vi "findChannelIndexes.vi"(8 "error in (no error)":errorcluster, 10 "index":i32, 11 "ScriptEventList in":refnum<class "ScriptEventList.lvclass">) -> (0 "error out":errorcluster, 1 "noneFound":bool, 2 "indexArray":i32[](array[numeric]), 3 "ScriptEventList out":refnum<class "ScriptEventList.lvclass">)   [LabVIEW 2009, in "Tools.lvlib" / "Scripting.lvlib" / "ScriptEventList.lvclass"]
uses:
  ScriptEventList.lvclass
  ScriptEventList.lvclass/ScriptEventList.ctl
  ScriptEvent.lvclass
  DatabaseHelpers/Database Objects/Channel/Channel.lvclass
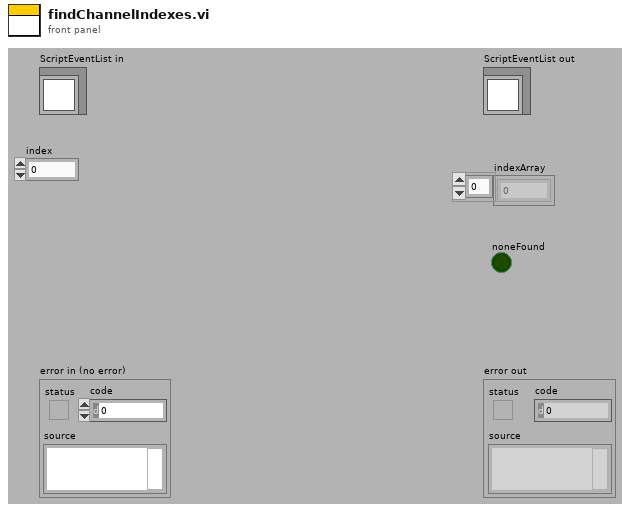
[diagram p1: front panel]
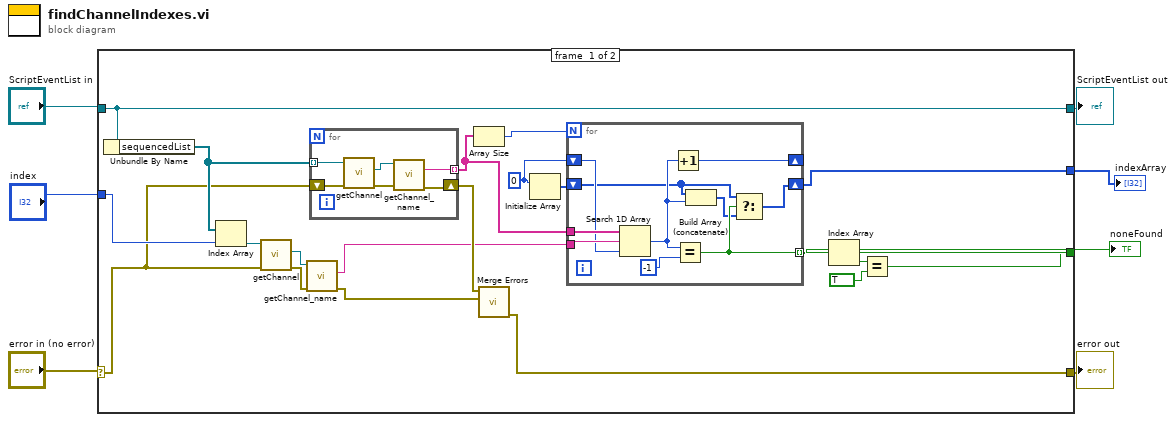
[diagram p0: block diagram]
diagram:
  n1 = case shown="No Error" "error in (no error)" {
    selector: "error in (no error)" -> [w21 w45]
    tunnel: [w23 w45] -> w1
    tunnel: [w27 w44] -> w4
    tunnel: "ScriptEventList in" -> [w27 w44]
    tunnel: "index" -> [w25 _]
    tunnel: [w8 _] -> w3
    tunnel: [w9 _] -> w2
    frame #0 {
      w13 = 0
      n2 = Unbundle By Name(w27) -> ("sequencedList"=w26:refnum<class "ScriptEvent.lvclass">[])
      n3 = Index Array(array=w26, index=w25) -> (element=w22:refnum<class "ScriptEvent.lvclass">)
      n4 = call-dynamic "getChannel.vi"("error in (no error)"=w21, "ScriptEvent.lvclass in"=w22) -> ("error out"=w20:errorcluster, "Channel.lvclass"=w18:refnum<class "Channel.lvclass">)  [unwired: 7 in, 1 out]
      n5 = call "getChannel_name.vi"("error in (no error)"=w20, "Channel.lvclass in"=w18) -> ("error out"=w19:errorcluster, "channel_name"=w15:string)  [unwired: 7 in, 1 out]
      n6 = for {
        tunnel: w26 -> [w41] mode=indexing
        tunnel: [w39] -> w16 mode=indexing
        shift-right: [w38] -> w24
        shift-left: w21 -> [w40]
        n7 = call-dynamic "getChannel.vi"("error in (no error)"=w40, "ScriptEvent.lvclass in"=w41) -> ("error out"=w43:errorcluster, "Channel.lvclass"=w42:refnum<class "Channel.lvclass">)  [unwired: 7 in, 1 out]
        n8 = call "getChannel_name.vi"("error in (no error)"=w43, "Channel.lvclass in"=w42) -> ("error out"=w38:errorcluster, "channel_name"=w39:string)  [unwired: 7 in, 1 out]
      }
      n9 = Array Size(array=w16) -> (size(s)=w17:i32)
      n10 = call <vilib>:"Merge Errors.vi"("error in 2 (no error)"=w19, "error in 1 (no error)"=w24) -> ("error out"=w23:errorcluster)  [unwired: 5 in]
      n11 = Initialize Array(w13) -> (w14:i32[])  [unwired: 1 in]
      n12 = for {
        N: w17 -> [_]
        tunnel: w16 -> [w37]
        tunnel: w15 -> [w36]
        shift-right: [w33] -> _
        shift-left: w13 -> [w34]
        tunnel: [w32] -> w10 mode=indexing
        shift-right: [w29] -> w8
        shift-left: w14 -> [w28]
        n13 = Search 1D Array(1D array=w37, element=w36, start index (0)=w34) -> (index of element=w31:i32)
        n14 = Increment(x=w31) -> (x+1=w33:i32)
        n15 = Equal?(x=w31, y=-1) -> (x = y?=w32:bool)
        n16 = Build Array (concatenate)(w28, w31) -> (w30:i32[])
        n17 = Select(t=w28, s=w32, f=w30) -> (s? t:f=w29:i32[])
      }
      n18 = Index Array(array=w10) -> (element=w12:bool)  [unwired: 1 in]
      n19 = Equal?(x=w12, y=TRUE) -> (x = y?=w9:bool)
    }
    frame #1 {
    }
  }
  "error out" <- w1
  "ScriptEventList out" <- w4
  "noneFound" <- w2
  "indexArray" <- w3
